vi "String to Word Integer.vi"(6 "string":string) -> (2 "Integer":i16)   [LabVIEW 2011]
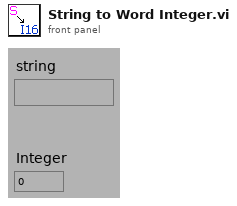
[diagram p1: front panel]
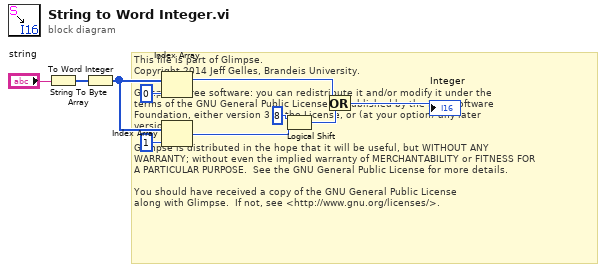
[diagram p0: block diagram]
diagram:
  # "This file is part of Glimpse. \nCopyright 2014 Jeff Gelles, Brandeis University.    \n\nGlimpse is free software: you can redistribute it and/or modify it under the \nterms of the GNU General Public License as published by the Free Software \nFoundation, either version 3 of the License, or (at your option) any later \nversion.\n\nGlimpse is distributed in the hope that it will be useful, but WITHOUT ANY \nWARRANTY; without even the implied warranty of MERCHANTABILITY or FITNESS FOR \nA PARTICULAR PURPOSE.  See the GNU General Public License for more details.\n\nYou should have received a copy of the GNU General Public License\nalong with Glimpse.  If not, see <http://www.gnu.org/licenses/>."
  n1 = String To Byte Array(string="string") -> (unsigned byte array=w10:u8[])
  n2 = To Word Integer(number=w10) -> (16bit integer=w4:i16[])
  n3 = Index Array(array=w4, index=0) -> (element=w3:i16)
  n4 = Index Array(array=w4, index=1) -> (element=w2:i16)
  n5 = Logical Shift(y=i16 8, x=w2) -> (x << y=w8:i16)
  n6 = Or(x=w3, y=w8) -> (x .or. y?=→"Integer":i16)
